vi "CTL_Simulate Resistor.vi"(6 "error in (no error)":errorcluster, 9 "Level IN inches":dbl, 10 "ChB Spec Range":T1, 11 "ChA Spec Range":T1) -> (2 "Ch B  Ohms":dbl, 3 "Ch A  Ohms":dbl, 4 "error out":errorcluster)   [LabVIEW 2024]
uses:
  Control Definitions/Def Spec Range.ctl
panel:
  # "Ch(n) HI \n\nCh(n)Lo    \n\nCh(n+1)Hi    \n\nR Hi      \nR Lo"
  # "Ch(n) HI \n\nCh(n)Lo    \n\nCh(n+1)Hi    \n\nR Hi      \nR Lo"
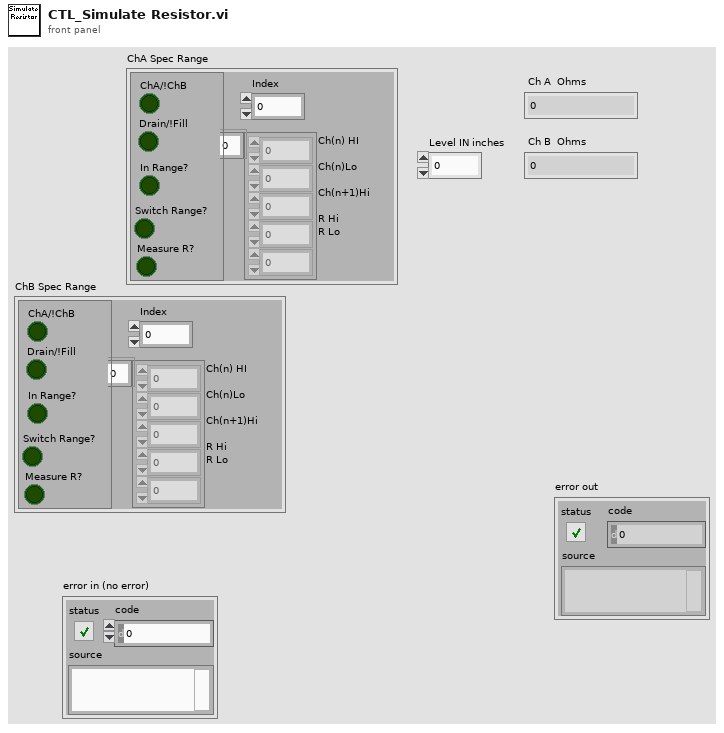
[diagram p1: front panel]
types:
  T1 = typedef "Def Spec Range.ctl" = cluster{cluster{"ChA/!ChB":bool, "Drain/!Fill":bool, "In Range?":bool, "Switch Range?":bool, "Measure R?":bool}, "Index":i32, dbl[]}
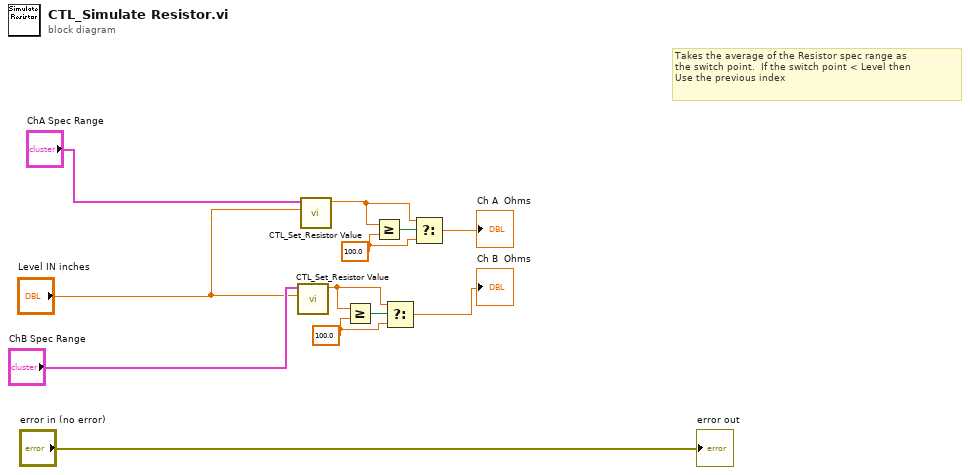
[diagram p0: block diagram]
diagram:
  w3 = 100.0 ("y")
  w5 = 100.0 ("y")
  # "Takes the average of the Resistor spec range as \nthe switch point.  If the switch point < Level then \nUse the previous index"
  n1 = call "CTL_Set_Resistor Value.vi"("Level IN inches"="Level IN inches", "ChA Spec Range"="ChB Spec Range") -> ("Numeric"=w8:dbl)  [unwired: 9 in]
  n2 = call "CTL_Set_Resistor Value.vi"("Level IN inches"="Level IN inches", "ChA Spec Range"="ChA Spec Range") -> ("Numeric"=w2:dbl)  [unwired: 9 in]
  n3 = Greater Or Equal?(x=w8, y=w5) -> (x >= y?=w6:bool)
  n4 = Greater Or Equal?(x=w2, y=w3) -> (x >= y?=w4:bool)
  n5 = Select(t=w8, s=w6, f=w5) -> (s? t:f=→"Ch B  Ohms":dbl)
  n6 = Select(t=w2, s=w4, f=w3) -> (s? t:f=→"Ch A  Ohms":dbl)
  "error out" <- "error in (no error)"
